vi "运维调试_CODCr.vi"() -> ()   [LabVIEW 2016, in "CodCr.lvlib"]
uses:
  CodCr.lvlib
  <vilib>/Utility/miscctls.llb/LVPointTypeDef.ctl
  <vilib>/Plasmionique/MB Master/MB_Master_Serial/MB_Master_Serial.lvclass
  C:/Program Files (x86)/National Instruments/LabVIEW 2016/vi.lib/Plasmionique/MB Master/MB_Master/MB_Master.lvclass
  <vilib>/Plasmionique/MB Master/MB Master.lvlib
  <vilib>/ptbypt/NI_PtbyPt.lvlib
panel:
  out "source":string
  in  "标样核查":bool
  out "启动时间":timestamp format="%<%Y/%m/%d %H:%M:%S>T"
  out "主循环次数":i32
  out "status":bool
  out "启动测量模式":T1(ring)
  out "曲线斜率B":sgl
  out "曲线斜率K":sgl
  out "量程上限":sgl
  out "量程下限":sgl
  out "消解时长":u16
  out "消解温度":u16
  out "测量精度":u16
  out "测量结果":sgl
  out "标样参考值":sgl
  out "量程":u16
  out "工作状态":T1(ring)
  out "仪器时间":timestamp format="%<%X\n%x>T"
  out "关键参数区":T2
  out "状态告警区":T3
  out "测量数据区":T4 {"单位" items=["ug/L", "mg/L", "ppm", "mg/m3", "cm", "ppb", "ug/m3", "%", "nmol/mol", "umol/mol", "MPN/L", "MPN/100ml", "ng/m3", "NTU", "无量纲", "ms/cm", "us/cm", "℃", "mV", "万个/L"]}
  out "系统时间":timestamp format="%<%Y/%m/%d %H:%M:%S>T"
  in  "VISA Resource":refnum<visa-resource-name>="COM9"
  out "Registers":u16[](array[numeric])
  in  "枚举":enum16{"读取", "写入", "读取参数"}(ring)
  in  "停止":bool
  in  "校时":bool
  in  "标样校准":bool
  in  "空白校准":bool
  in  "零点核查":bool
  in  "跨度核查":bool
  in  "水样测试":bool
  in  "返回":bool
  in  "设置":bool
  # "mg/L"
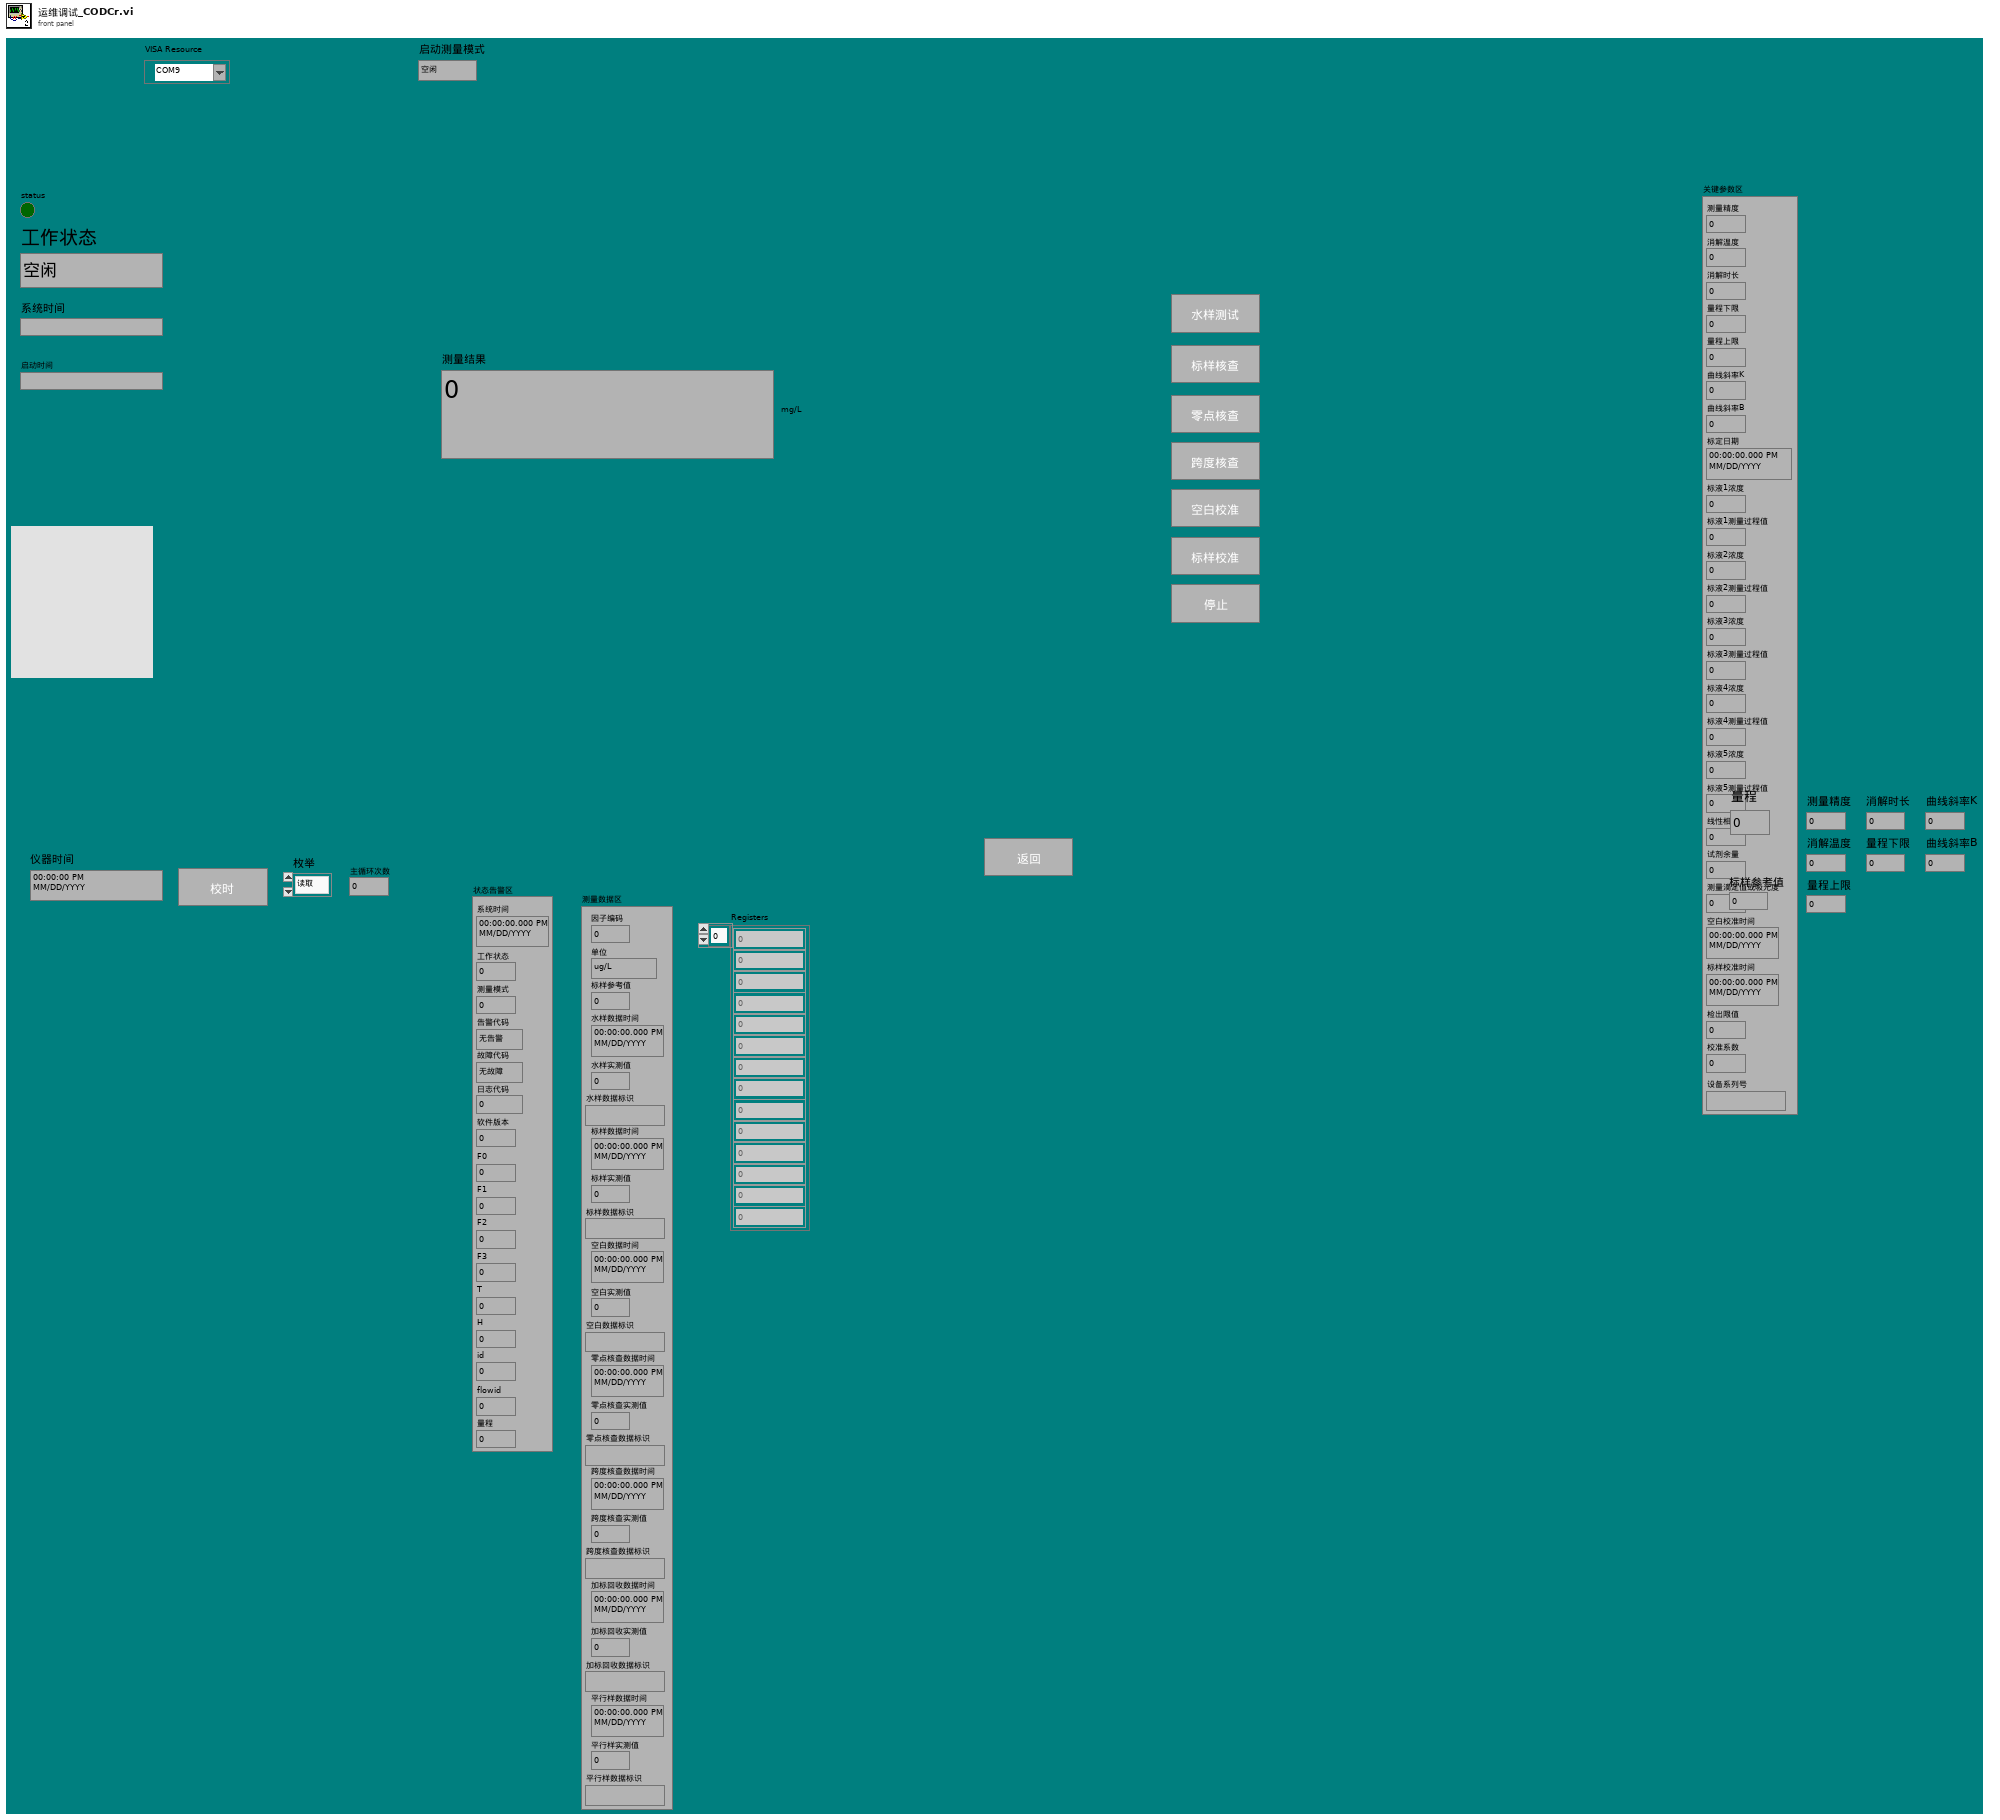
[diagram p1: front panel]
types:
  T1 = enum16{"空闲", "水样测试", "标样核查", "零点核查", "跨度核查", "空白测试", "平行样测试", "加标回收", "空白校准", "标样校准", "初始化（清洗）"}
  T2 = cluster{"测量精度":u16, "消解温度":u16, "消解时长":u16, "量程下限":sgl, "量程上限":sgl, "曲线斜率K":sgl, "曲线斜率B":sgl, "标定日期":timestamp, "标液1浓度":sgl, "标液1测量过程值":sgl, "标液2浓度":sgl, "标液2测量过程值":sgl, "标液3浓度":sgl, "标液3测量过程值":sgl, "标液4浓度":sgl, "标液4测量过程值":sgl, "标液5浓度":sgl, "标液5测量过程值":sgl, "线性相关系数":sgl, "试剂余量":u32, "测量滴定值或吸光度":sgl, "空白校准时间":timestamp, "标样校准时间":timestamp, "检出限值":sgl, "校准系数":sgl, "设备系列号":string}
  T3 = cluster{"系统时间":timestamp, "工作状态":u16, "测量模式":u16, "告警代码":enum16{"无告警", "缺试剂告警", "缺水样告警", "缺蒸馏水告警", "缺标液告警", "仪表漏液告警", "标定异常告警", "超量程告警", "加热异常", "低试剂预警", "超上限告警", "超下限告警", "仪表内部其他异常", "滴定异常告警", "电极异常告警", "量程切换告警", "参数设置告警", "PH电极电位异常", "电导率电极异常", "浊度光度异常", "溶解氧电极异常", "溶解氧光强异常", "温度异常告警", "PH异常告警", "溶解氧异常告警", "电导率异常告警", "浊度异常告警", "叶绿素异常告警", "藻密度异常告警", "蓝绿藻异常告警", "ORP异常告警", "氨氮异常告警", "清洁刷异常告警", "SD卡异常告警", "蓝牙异常告警", "Wifi异常告警", "流程异常告警"}, "故障代码":enum16{"无故障", "电机故障", "温度故障", "通讯故障", "滴定故障"}, "日志代码":u16, "软件版本":u16, "F0":sgl, "F1":sgl, "F2":sgl, "F3":sgl, "T":sgl, "H":sgl, "id":u16, "flowid":u16, "量程":u16}
  T4 = cluster{"因子编码":u32, "单位":u16, "标样参考值":sgl, "水样数据时间":timestamp, "水样实测值":sgl, "水样数据标识":string, "标样数据时间":timestamp, "标样实测值":sgl, "标样数据标识":string, "空白数据时间":timestamp, "空白实测值":sgl, "空白数据标识":string, "零点核查数据时间":timestamp, "零点核查实测值":sgl, "零点核查数据标识":string, "跨度核查数据时间":timestamp, "跨度核查实测值":sgl, "跨度核查数据标识":string, "加标回收数据时间":timestamp, "加标回收实测值":sgl, "加标回收数据标识":string, "平行样数据时间":timestamp, "平行样实测值":sgl, "平行样数据标识":string}
  T5 = cluster{"baud rate (bps)":u32, "stop bits":u16, "parity":u16, "flow control":u16, "timeout":u32, "retries":i32}
  T6 = cluster{"starting address":u16, "number of holding registers":u16}
  T7 = typedef "LVPointTypeDef.ctl" = cluster{"Horizontal":i16, "Vertical":i16}
  T8 = cluster{"时间标识":timestamp, "监测值":sgl, "单位":u16, "数据标识":string, "因子编码":u32, "标样参考值":sgl, "F0":sgl, "F1":sgl, "F2":sgl, "F3":sgl, "温度":sgl, "湿度":sgl, "量程标识":string}
  T9 = cluster{"系统时间":timestamp, "工作状态":enum16{"空闲", "水样测试", "标样核查", "零点核查", "跨度核查", "空白测试", "平行样测试", "加标回收", "空白校准", "标样校准", "初始化（清洗）"}, "测量模式":enum16{"待机", "连续模式", "周期模式", "定点模式", "受控模式", "手动模式"}, "告警代码":enum16{"无告警", "缺试剂告警", "缺水样告警", "缺蒸馏水告警", "缺标液告警", "仪表漏液告警", "标定异常告警", "超量程告警", "加热异常", "低试剂预警", "超上限告警", "超下限告警", "仪表内部其他异常", "滴定异常告警", "电极异常告警", "量程切换告警", "参数设置告警", "PH电极电位异常", "电导率电极异常", "浊度光度异常", "溶解氧电极异常", "溶解氧光强异常", "温度异常告警", "PH异常告警", "溶解氧异常告警", "电导率异常告警", "浊度异常告警", "叶绿素异常告警", "藻密度异常告警", "蓝绿藻异常告警", "ORP异常告警", "氨氮异常告警", "清洁刷异常告警", "SD卡异常告警", "蓝牙异常告警", "Wifi异常告警", "流程异常告警"}, "故障代码":enum16{"无故障", "电机故障", "温度故障", "通讯故障", "滴定故障"}, "日志代码":u16, "软件版本":u16, "F0":sgl, "F1":sgl, "F2":sgl, "F3":sgl, "T":sgl, "H":sgl, "id":u16, "flowid":u16, "量程":u16}
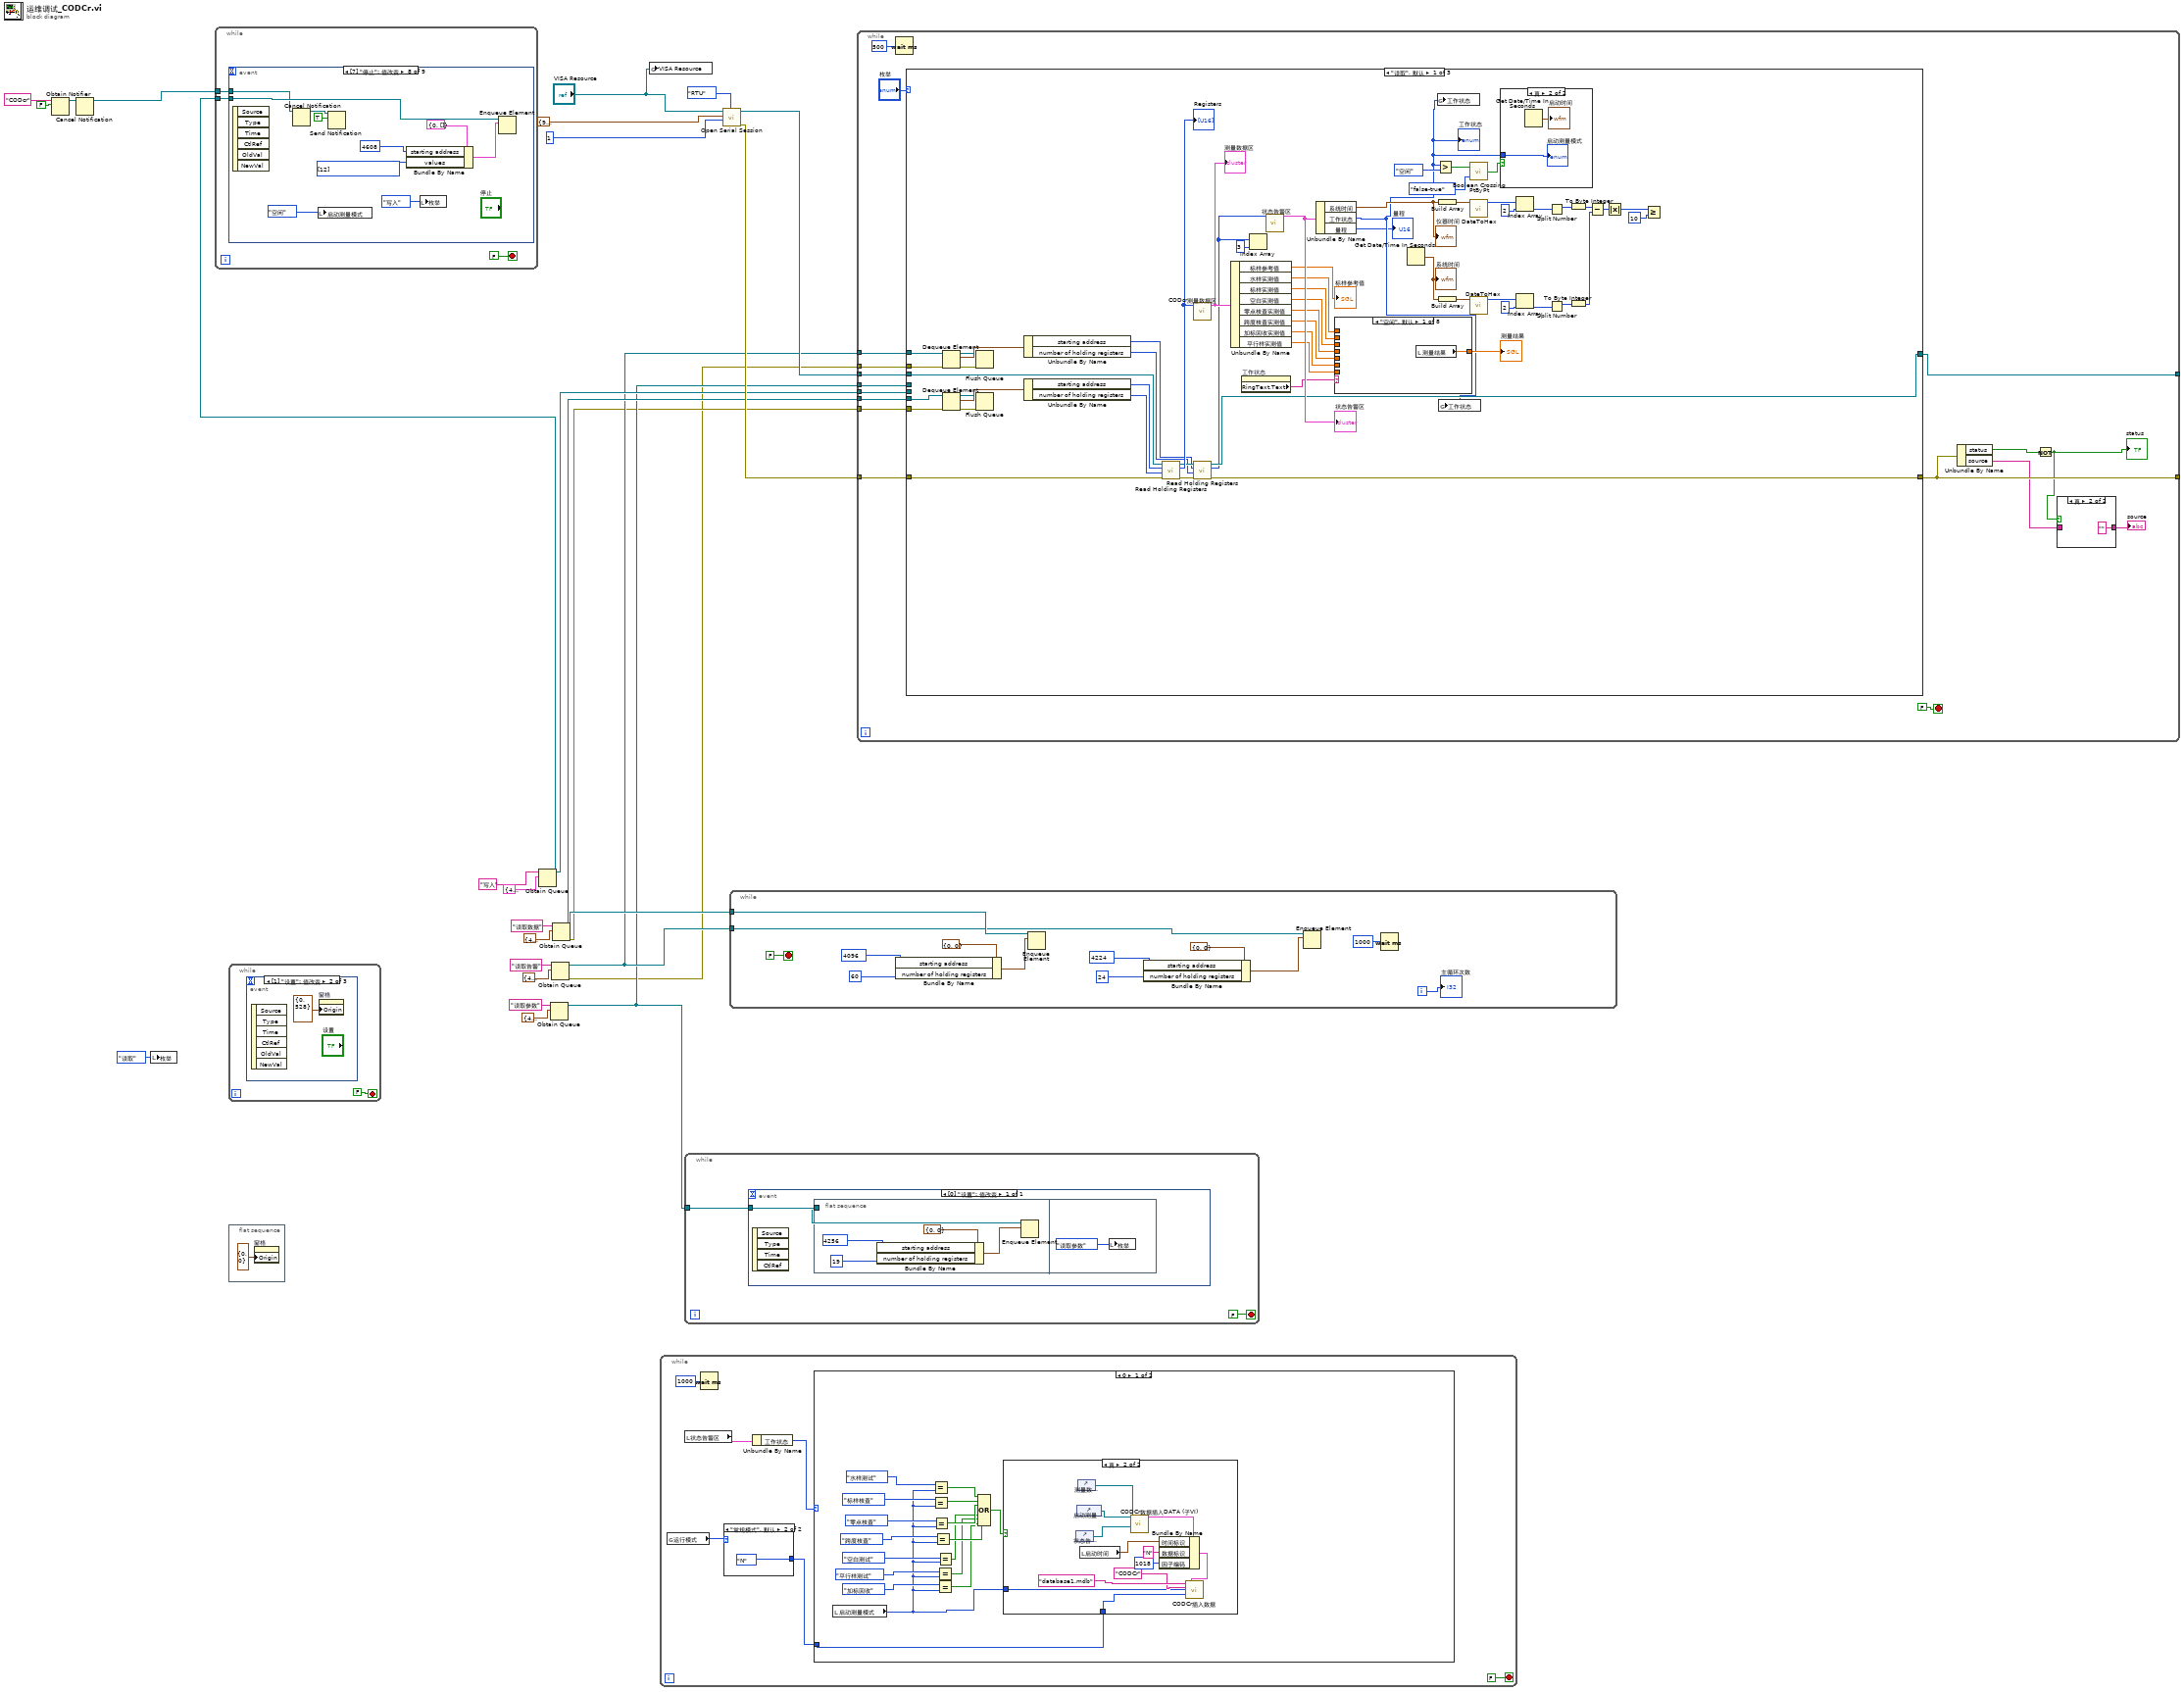
[diagram p0: block diagram]
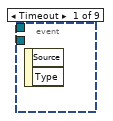
[diagram p2: hidden frame]
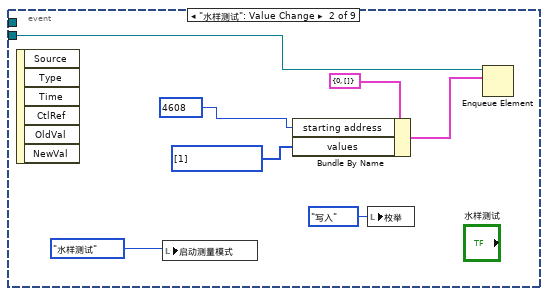
[diagram p3: hidden frame]
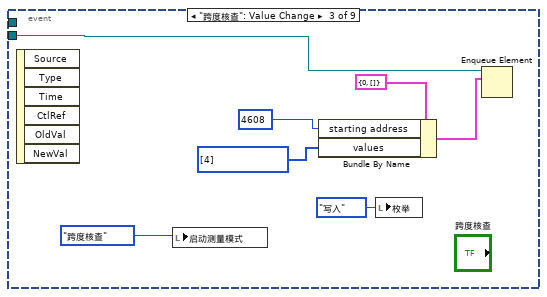
[diagram p4: hidden frame]
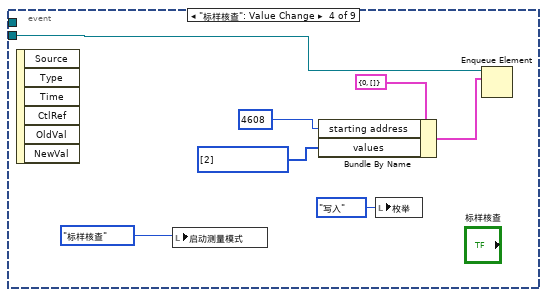
[diagram p5: hidden frame]
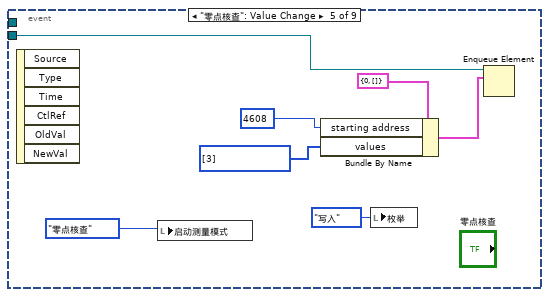
[diagram p6: hidden frame]
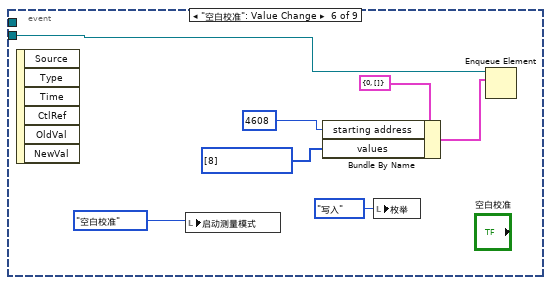
[diagram p7: hidden frame]
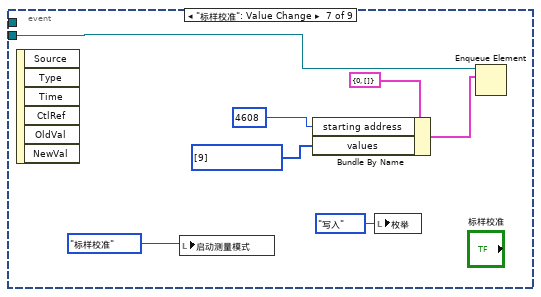
[diagram p8: hidden frame]
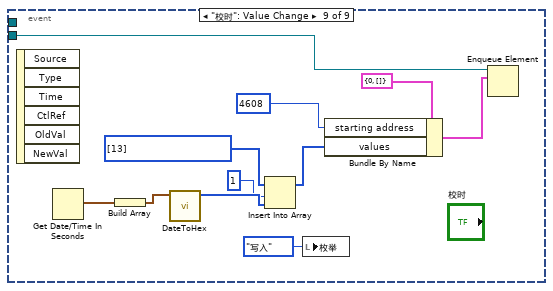
[diagram p9: hidden frame]
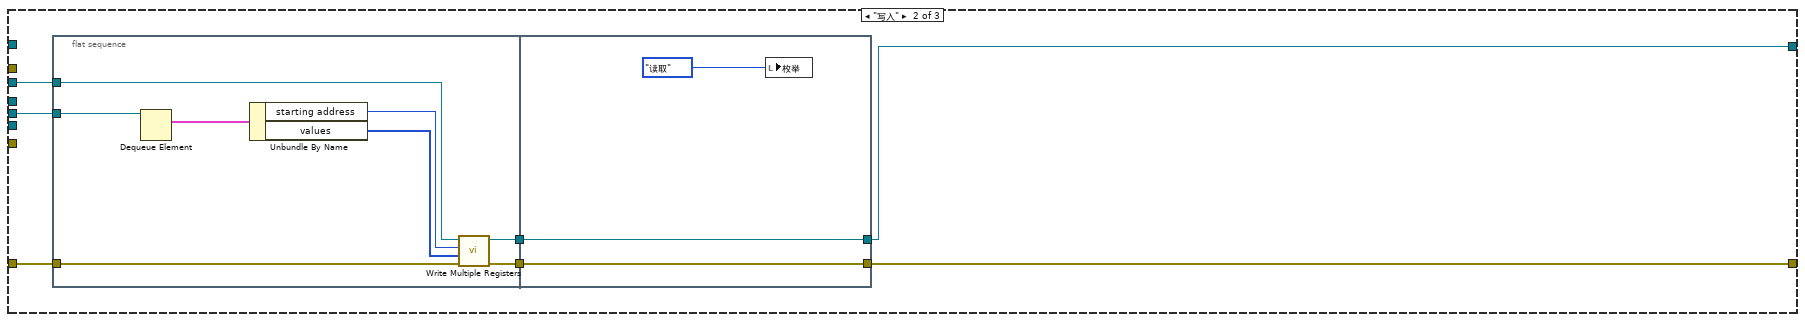
[diagram p19: hidden frame]
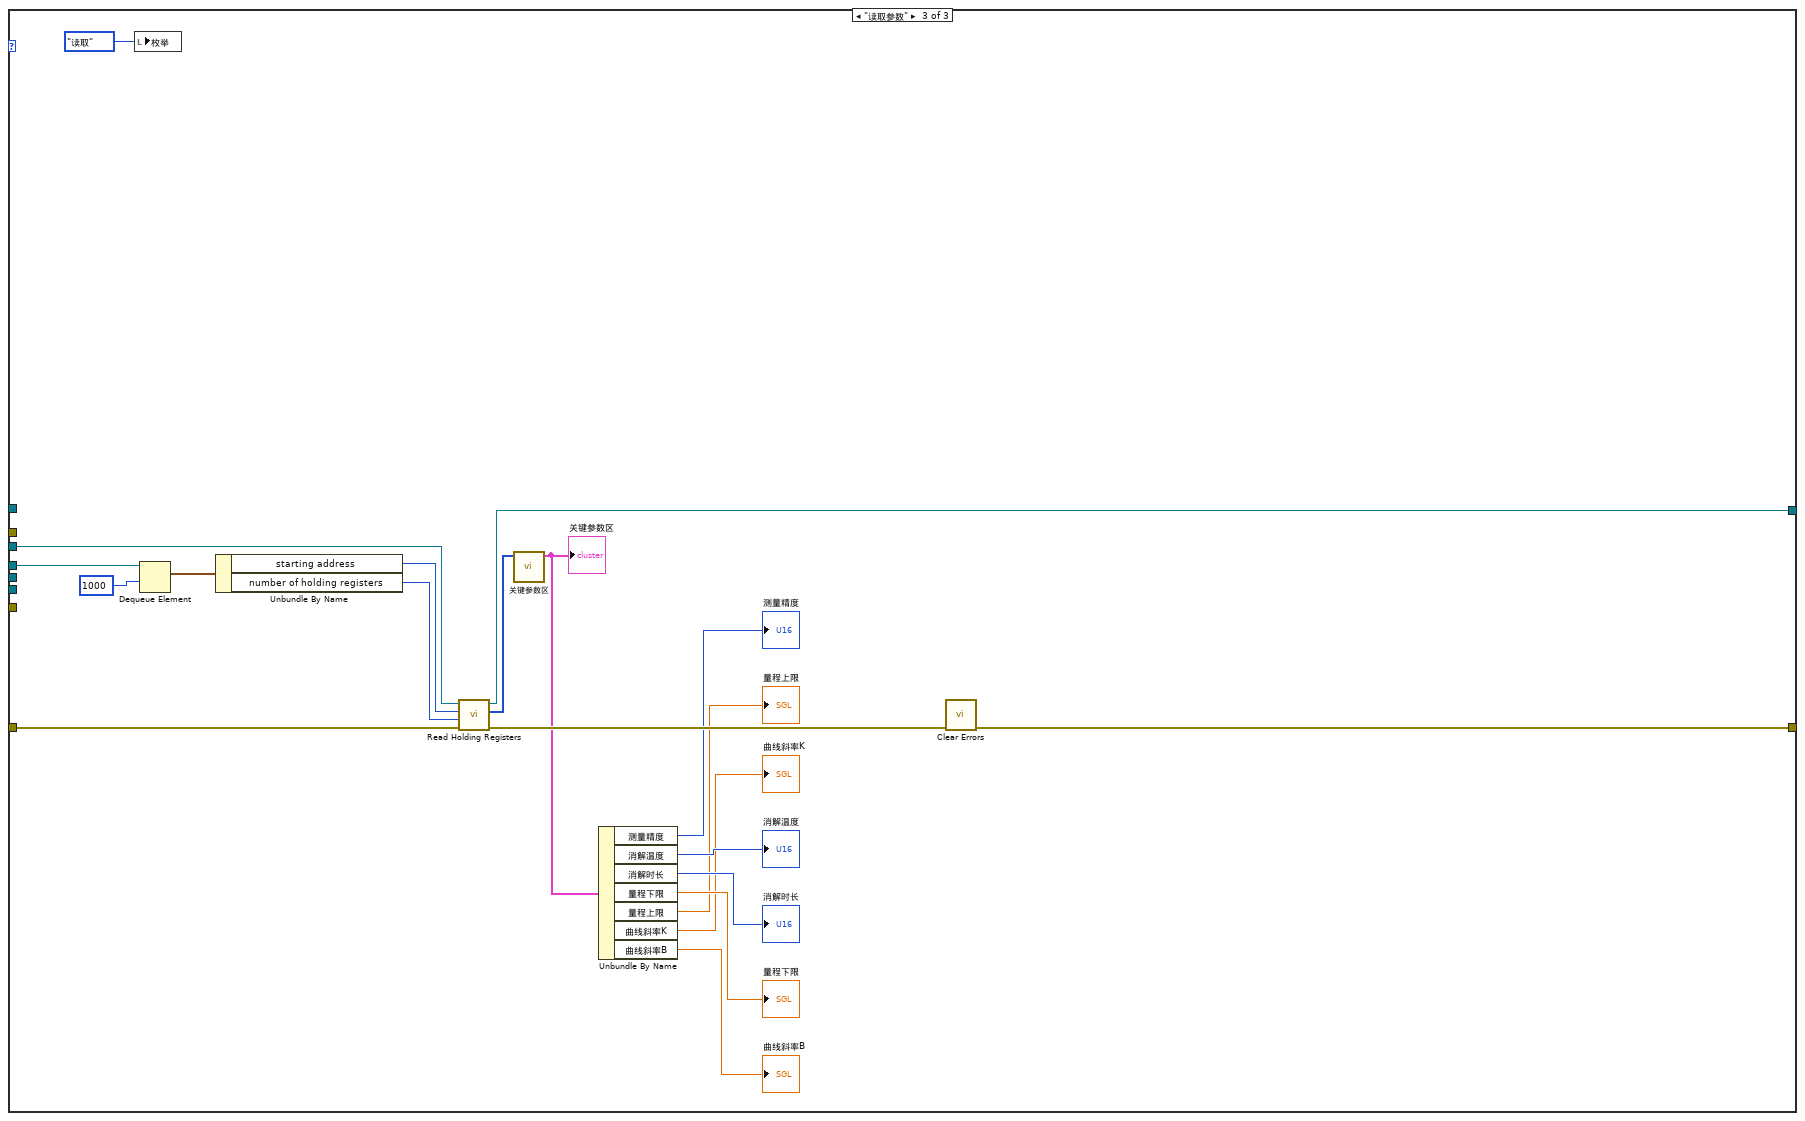
[diagram p20: hidden frame]
diagram:
  n1 = Obtain Notifier(name (unnamed)="CODcr" ("名称（未命名）"), notification data type=FALSE) -> (notifier out=w2:refnum<notifier>)  [unwired: 2 in, 2 out]
  n2 = Cancel Notification(0:w2) -> (8:w3:refnum<notifier>)  [unwired: 1 in, 2 out]
  n3 = local write "枚举"(enum16{"读取", "写入", "读取参数"}."读取" ("枚举")) -> ()
  n4 = while {
    stop <- FALSE stop-if-true
    n5 = event shown="[1] \"设置\": 值改变" {
      selector: _ -> [_ _ _]
      dyn-events: _ -> [_ _ _]
      timeout: _ -> [_ _ _]
      event Timeout {
        n6 = event-data() -> ()  [unwired: 1 in, 3 out]
      }
      event "设置": Value Change {
        n7 = event-data() -> ()  [unwired: 1 in, 6 out]
        n8 = property on="窗格" class="Pane"("Origin"=T7 {"Horizontal"=0, "Vertical"=528} ("原点")) -> ()  [unwired: 2 in, 2 out]
      }
      event "返回": Value Change {
        n9 = event-data() -> ()  [unwired: 1 in, 6 out]
        n10 = property on="窗格" class="Pane"("Origin"=T7 {"Horizontal"=0, "Vertical"=0} ("原点")) -> ()  [unwired: 2 in, 2 out]
      }
    }
  }
  n11 = flat-sequence {
    frame #0 {
      n12 = property on="窗格" class="Pane"("Origin"=T7 {"Horizontal"=0, "Vertical"=0} ("原点")) -> ()  [unwired: 2 in, 2 out]
    }
  }
  n13 = Obtain Queue(name (unnamed)="写入" ("名称（未命名）"), element data type=cluster{"starting address":u16, "values":u16[]} {"starting address"=4096, "values"=[]}) -> (queue out=w15:refnum<queue>)  [unwired: 3 in, 2 out]
  n14 = while {
    tunnel: w15 -> [w31]
    tunnel: w3 -> [w30]
    stop <- FALSE stop-if-true
    n15 = event shown="[7] \"停止\": 值改变" {
      selector: _ -> [_ _ _ _ _ _ _ _ _]
      dyn-events: _ -> [_ _ _ _ _ _ _ _ _]
      timeout: _ -> [_ _ _ _ _ _ _ _ _]
      tunnel: w31 -> [_ w39 w42 w49 w56 w63 w70 w80 w92]
      tunnel: w30 -> [_ _ _ _ _ _ _ w78 _]
      event Timeout {
        n16 = event-data() -> ()  [unwired: 1 in, 2 out]
      }
      event "水样测试": Value Change {
        n17 = event-data() -> ()  [unwired: 1 in, 6 out]
        n18 = local write "启动测量模式"(T1."水样测试" ("启动测量模式")) -> ()
        n19 = Bundle By Name(cluster=cluster{"starting address":u16, "values":u16[]} {"starting address"=0, "values"=[]} ("元素"), "starting address"=u16 4608, "values"=u16[] [1]) -> (w37:cluster{"starting address":u16, "values":u16[]})
        n20 = local write "枚举"(enum16{"读取", "写入", "读取参数"}."写入" ("枚举")) -> ()
        n21 = Enqueue Element(queue=w39, element=w37) -> ()  [unwired: 2 in, 3 out]
      }
      event "跨度核查": Value Change {
        n22 = event-data() -> ()  [unwired: 1 in, 6 out]
        n23 = local write "启动测量模式"(T1."跨度核查" ("启动测量模式")) -> ()
        n24 = Bundle By Name(cluster=cluster{"starting address":u16, "values":u16[]} {"starting address"=0, "values"=[]} ("元素"), "starting address"=u16 4608, "values"=u16[] [4]) -> (w45:cluster{"starting address":u16, "values":u16[]})
        n25 = local write "枚举"(enum16{"读取", "写入", "读取参数"}."写入" ("枚举")) -> ()
        n26 = Enqueue Element(queue=w42, element=w45) -> ()  [unwired: 2 in, 3 out]
      }
      event "标样核查": Value Change {
        n27 = event-data() -> ()  [unwired: 1 in, 6 out]
        n28 = local write "启动测量模式"(T1."标样核查" ("启动测量模式")) -> ()
        n29 = Bundle By Name(cluster=cluster{"starting address":u16, "values":u16[]} {"starting address"=0, "values"=[]} ("元素"), "starting address"=u16 4608, "values"=u16[] [2]) -> (w52:cluster{"starting address":u16, "values":u16[]})
        n30 = local write "枚举"(enum16{"读取", "写入", "读取参数"}."写入" ("枚举")) -> ()
        n31 = Enqueue Element(queue=w49, element=w52) -> ()  [unwired: 2 in, 3 out]
      }
      event "零点核查": Value Change {
        n32 = event-data() -> ()  [unwired: 1 in, 6 out]
        n33 = local write "启动测量模式"(T1."零点核查" ("启动测量模式")) -> ()
        n34 = Bundle By Name(cluster=cluster{"starting address":u16, "values":u16[]} {"starting address"=0, "values"=[]} ("元素"), "starting address"=u16 4608, "values"=u16[] [3]) -> (w59:cluster{"starting address":u16, "values":u16[]})
        n35 = local write "枚举"(enum16{"读取", "写入", "读取参数"}."写入" ("枚举")) -> ()
        n36 = Enqueue Element(queue=w56, element=w59) -> ()  [unwired: 2 in, 3 out]
      }
      event "空白校准": Value Change {
        n37 = event-data() -> ()  [unwired: 1 in, 6 out]
        n38 = local write "启动测量模式"(T1."空白校准" ("启动测量模式")) -> ()
        n39 = Bundle By Name(cluster=cluster{"starting address":u16, "values":u16[]} {"starting address"=0, "values"=[]} ("元素"), "starting address"=u16 4608, "values"=u16[] [8]) -> (w66:cluster{"starting address":u16, "values":u16[]})
        n40 = local write "枚举"(enum16{"读取", "写入", "读取参数"}."写入" ("枚举")) -> ()
        n41 = Enqueue Element(queue=w63, element=w66) -> ()  [unwired: 2 in, 3 out]
      }
      event "标样校准": Value Change {
        n42 = event-data() -> ()  [unwired: 1 in, 6 out]
        n43 = local write "启动测量模式"(T1."标样校准" ("启动测量模式")) -> ()
        n44 = Bundle By Name(cluster=cluster{"starting address":u16, "values":u16[]} {"starting address"=0, "values"=[]} ("元素"), "starting address"=u16 4608, "values"=u16[] [9]) -> (w73:cluster{"starting address":u16, "values":u16[]})
        n45 = local write "枚举"(enum16{"读取", "写入", "读取参数"}."写入" ("枚举")) -> ()
        n46 = Enqueue Element(queue=w70, element=w73) -> ()  [unwired: 2 in, 3 out]
      }
      event "停止": Value Change {
        n47 = event-data() -> ()  [unwired: 1 in, 6 out]
        n48 = Cancel Notification(0:w78) -> (8:w77:refnum<notifier>)  [unwired: 1 in, 2 out]
        n49 = local write "启动测量模式"(T1."空闲" ("启动测量模式")) -> ()
        n50 = Send Notification(notification=TRUE ("通知"), notifier=w77) -> ()  [unwired: 1 in, 2 out]
        n51 = Bundle By Name(cluster=cluster{"starting address":u16, "values":u16[]} {"starting address"=0, "values"=[]} ("元素"), "starting address"=u16 4608, "values"=u16[] [12]) -> (w83:cluster{"starting address":u16, "values":u16[]})
        n52 = local write "枚举"(enum16{"读取", "写入", "读取参数"}."写入" ("枚举")) -> ()
        n53 = Enqueue Element(queue=w80, element=w83) -> ()  [unwired: 2 in, 3 out]
      }
      event "校时": Value Change {
        n54 = event-data() -> ()  [unwired: 1 in, 6 out]
        n55 = Get Date/Time In Seconds() -> (seconds since 1Jan1904=w91:timestamp)
        n56 = Build Array(w91) -> (w90:timestamp[])
        n57 = call "DateToHex.vi"("DATE"=w90) -> ("数组"=w88:u16[])  [unwired: 10 in]
        n58 = Insert Into Array(array=u16[] [13] ("values"), index=1 ("索引"), new element=w88) -> (w86:u16[])
        n59 = local write "枚举"(enum16{"读取", "写入", "读取参数"}."写入" ("枚举")) -> ()
        n60 = Bundle By Name(cluster=cluster{"starting address":u16, "values":u16[]} {"starting address"=0, "values"=[]} ("元素"), "starting address"=u16 4608, "values"=w86) -> (w94:cluster{"starting address":u16, "values":u16[]})
        n61 = Enqueue Element(queue=w92, element=w94) -> ()  [unwired: 2 in, 3 out]
      }
    }
  }
  n62 = Obtain Queue(name (unnamed)="读取参数" ("名称（未命名）"), element data type=T6 {"starting address"=4096, "number of holding registers"=100}) -> (queue out=w9:refnum<queue>)  [unwired: 3 in, 2 out]
  n63 = Obtain Queue(name (unnamed)="读取告警" ("名称（未命名）"), element data type=T6 {"starting address"=4096, "number of holding registers"=100}) -> (queue out=w12:refnum<queue>, error out=w6:errorcluster)  [unwired: 3 in, 1 out]
  n64 = Obtain Queue(name (unnamed)="读取数据" ("名称（未命名）"), element data type=T6 {"starting address"=4096, "number of holding registers"=100}) -> (queue out=w16:refnum<queue>, error out=w7:errorcluster)  [unwired: 3 in, 1 out]
  n65 = global write "CODcr全局变量.vi" "VISA Resource"("VISA Resource") -> ()
  n66 = while {
    stop <- FALSE stop-if-true
    n67 = global read "系统变量.vi" "运行模式"() -> (w97:enum16{"维护模式", "常规模式", "应急模式", "质控模式"})
    n68 = local read "状态告警区"() -> (w99:T3)
    n69 = Wait (ms)(milliseconds to wait=u32 1000 ("等待时间（毫秒）")) -> ()  [unwired: 1 out]
    n70 = case shown="\"常规模式\", 默认" w97 {
      tunnel: [enum16{"N", "M"}."M" ("数据类型") enum16{"N", "M"}."N" ("数据类型")] -> w96
      frame "维护模式" {
      }
      frame "常规模式", Default {
      }
    }
    n71 = Unbundle By Name(w99) -> ("工作状态"=w98:u16)
    n72 = case shown="0" w98 {
      tunnel: w96 -> [w120 _]
      frame 0 {
        n73 = local read "启动测量模式"() -> (w112:T1)
        n74 = Equal?(x=T1."水样测试" ("启动测量模式"), y=w112) -> (x = y?=w111:bool)
        n75 = Equal?(x=T1."标样核查" ("启动测量模式"), y=w112) -> (x = y?=w110:bool)
        n76 = Equal?(x=T1."零点核查" ("启动测量模式"), y=w112) -> (x = y?=w109:bool)
        n77 = Equal?(x=T1."跨度核查" ("启动测量模式"), y=w112) -> (x = y?=w108:bool)
        n78 = Equal?(x=T1."平行样测试" ("启动测量模式"), y=w112) -> (x = y?=w106:bool)
        n79 = Equal?(x=T1."加标回收" ("启动测量模式"), y=w112) -> (x = y?=w105:bool)
        n80 = Equal?(x=T1."空白测试" ("启动测量模式"), y=w112) -> (x = y?=w107:bool)
        n81 = Compound Arithmetic op=OR(w111, w110, w109, w108, w107, w106, w105) -> (w104:bool)
        n82 = case shown="真" w104 {
          tunnel: w112 -> [_ w130]
          tunnel: w120 -> [_ w129]
          frame False {
          }
          frame True {
            n83 = control-ref of="状态告警区"() -> (w126:refnum<vi>)
            n84 = control-ref of="启动测量模式"() -> (w128:refnum<vi>)
            n85 = control-ref of="测量数据区"() -> (w127:refnum<vi>)
            n86 = local read "启动时间"() -> (w124:timestamp)
            n87 = call "CODCr数据插入DATA (子VI).vi"("reference 2"=w126, "reference"=w127, "Enum输入"=w128) -> ("data"=w125:T8)  [unwired: 8 in]
            n88 = Bundle By Name(cluster=w125, "时间标识"=w124, "数据标识"="N", "因子编码"=u32 1018) -> (w123:T8)
            n89 = call "CODCr插入数据.vi"("database"="database1.mdb", "data"=w123, "table"="CODCr", "测量模式"=w130, "数据类型"=w129) -> ()  [unwired: 10 in, 1 out]
          }
        }
      }
      frame 1, Default {
      }
    }
  }
  n90 = while {
    tunnel: w9 -> [w133]
    stop <- FALSE stop-if-true
    n91 = event shown="[0] \"设置\": 值改变" {
      selector: _ -> [_]
      dyn-events: _ -> [_]
      timeout: _ -> [_]
      tunnel: w133 -> [w135]
      event "设置": Value Change {
        n92 = event-data() -> ()  [unwired: 1 in, 4 out]
        n93 = flat-sequence {
          tunnel: w135 -> [w136]
          frame #0 {
            n94 = Bundle By Name(cluster=T6 {"starting address"=0, "number of holding registers"=0} ("元素"), "starting address"=u16 4256, "number of holding registers"=u16 19) -> (w140:T6)
            n95 = Enqueue Element(queue=w136, element=w140) -> ()  [unwired: 2 in, 3 out]
          }
          frame #1 {
            n96 = local write "枚举"(enum16{"读取", "写入", "读取参数"}."读取参数" ("枚举")) -> ()
          }
        }
      }
    }
  }
  n97 = call <vilib>:"Open Serial Session.vi"("Mode (RTU)"=enum16{"RTU", "ASCII"}."RTU", "Slave ID"=u8 1, "Serial Config"=T5 {"baud rate (bps)"=9600, "stop bits"=10, "parity"=0, "flow control"=0, "timeout"=1000, "retries"=1}, "VISA Resource"="VISA Resource") -> ("Error out"=w24:errorcluster, "MB_Serial session"=w25:refnum<class "MB_Master_Serial.lvclass">)  [unwired: 6 in]
  n98 = while {
    tunnel: w16 -> [w152]
    tunnel: w12 -> [w143]
    i -> [w142]
    stop <- FALSE stop-if-true
    n99 = Bundle By Name(cluster=T6 {"starting address"=0, "number of holding registers"=0} ("元素"), "starting address"=u16 4096, "number of holding registers"=u16 60) -> (w150:T6)
    n100 = Enqueue Element(queue=w152, element=w150) -> ()  [unwired: 2 in, 3 out]
    n101 = Bundle By Name(cluster=T6 {"starting address"=0, "number of holding registers"=0} ("元素"), "starting address"=u16 4224, "number of holding registers"=u16 24) -> (w144:T6)
    n102 = Enqueue Element(queue=w143, element=w144) -> ()  [unwired: 2 in, 3 out]
    n103 = Wait (ms)(milliseconds to wait=u32 1000 ("等待时间（毫秒）")) -> ()  [unwired: 1 out]
    "主循环次数" <- w142
  }
  n104 = while {
    tunnel: w15 -> [w168]
    tunnel: w16 -> [w167]
    tunnel: w12 -> [w166]
    tunnel: w9 -> [w165]
    tunnel: w7 -> [w163]
    tunnel: w6 -> [w162]
    tunnel: w24 -> [w161]
    tunnel: [w159] -> _
    tunnel: w25 -> [w169]
    tunnel: [w164] -> _
    stop <- FALSE stop-if-true
    n105 = Wait (ms)(milliseconds to wait=u32 500 ("等待时间（毫秒）")) -> ()  [unwired: 1 out]
    n106 = case shown="\"读取\", 默认" "枚举" {
      tunnel: w169 -> [w231 w248 w271]
      tunnel: w161 -> [w206 w247 w270]
      tunnel: w168 -> [_ w246 _]
      tunnel: w167 -> [w230 _ _]
      tunnel: w166 -> [w225 _ _]
      tunnel: w165 -> [_ _ w272]
      tunnel: [w205 w242 w260] -> w159
      tunnel: [w187 w243 w261] -> w164
      tunnel: w163 -> [w181 _ _]
      tunnel: w162 -> [w178 _ _]
      frame "读取", Default {
        n107 = Dequeue Element(queue=w225, error in (no error)=w178) -> (queue out=w180:refnum<queue>, element=w224:T6, error out=w179:errorcluster)  [unwired: 1 in, 1 out]
        n108 = Dequeue Element(queue=w230, error in (no error)=w181) -> (queue out=w183:refnum<queue>, element=w229:T6, error out=w182:errorcluster)  [unwired: 1 in, 1 out]
        n109 = Flush Queue(queue=w180, error in (no error)=w179) -> ()  [unwired: 3 out]
        n110 = Flush Queue(queue=w183, error in (no error)=w182) -> ()  [unwired: 3 out]
        n111 = Unbundle By Name(w224) -> ("starting address"=w221:u16, "number of holding registers"=w220:u16)
        n112 = Unbundle By Name(w229) -> ("starting address"=w228:u16, "number of holding registers"=w227:u16)
        n113 = call <vilib>:"Read Holding Registers.vi"("error in (no error)"=w206, "quantity"=w227, "starting address"=w228, "MB session in"=w231) -> ("error out"=w222:errorcluster, "Registers"=w226:u16[], "MB session out"=w223:refnum<class "MB_Master_Serial.lvclass">)  [unwired: 5 in]
        "Registers" <- w226
        n114 = call "CODcr测量数据区.vi"("数组"=w226) -> ("测量数据区"=w218:T4)  [unwired: 10 in]
        "测量数据区" <- w218
        n115 = call <vilib>:"Read Holding Registers.vi"("error in (no error)"=w222, "quantity"=w220, "starting address"=w221, "MB session in"=w223) -> ("error out"=w205:errorcluster, "Registers"=w177:u16[], "MB session out"=w187:refnum<class "MB_Master_Serial.lvclass">)  [unwired: 5 in]
        n116 = Unbundle By Name(w218) -> ("标样参考值"=→"标样参考值":sgl, "水样实测值"=w214:sgl, "标样实测值"=w212:sgl, "空白实测值"=w209:sgl, "零点核查实测值"=w211:sgl, "跨度核查实测值"=w210:sgl, "加标回收实测值"=w207:sgl, "平行样实测值"=w208:sgl)
        n117 = property on="工作状态" class="Enum (严格)"() -> ("RingText.Text"=w215:string)  [unwired: 2 in, 2 out]
        n118 = Index Array(array=w177, index=3 ("索引")) -> ()  [unwired: 1 out]
        n119 = call "状态告警区.vi"("数组"=w177) -> ("状态告警区"=w219:T9)  [unwired: 10 in]
        "状态告警区" <- w219
        n120 = Unbundle By Name(w219) -> ("系统时间"=w188:timestamp, "工作状态"=w175:T1, "量程"=→"量程":u16)
        "仪器时间" <- w188
        "工作状态" <- w175
        n121 = case shown="\"空闲\", 默认" w215 {
          tunnel: w214 -> [_ w233 _ _ _ _ _ _]
          tunnel: [w232 w233 w234 w235 w236 w237 w238 w239] -> w213
          tunnel: w212 -> [_ _ w234 _ _ _ _ _]
          tunnel: w211 -> [_ _ _ w235 _ _ _ _]
          tunnel: w210 -> [_ _ _ _ w236 _ _ _]
          tunnel: w209 -> [_ _ _ _ _ w237 _ _]
          tunnel: w208 -> [_ _ _ _ _ _ w238 _]
          tunnel: w207 -> [_ _ _ _ _ _ _ w239]
          frame "空闲", Default {
            n122 = local read "测量结果"() -> (w232:sgl)
          }
          frame "水样测试" {
          }
          frame "标样核查" {
          }
          frame "零点核查" {
          }
          frame "跨度核查" {
          }
          frame "空白测试" {
          }
          frame "平行样测试" {
          }
          frame "加标回收" {
          }
        }
        "测量结果" <- w213
        n123 = Get Date/Time In Seconds() -> (seconds since 1Jan1904=w190:timestamp)
        "系统时间" <- w190
        n124 = Greater?(x=w175, y=T1."空闲") -> (0:w186:bool)
        n125 = global write "CODcr全局变量.vi" "工作状态"(w175) -> ()
        n126 = Build Array(w188) -> (w204:timestamp[])
        n127 = Build Array(w190) -> (w189:timestamp[])
        n128 = global write "CODCr工作状态.vi" "工作状态"(w175) -> ()
        n129 = call <vilib>:"Boolean Crossing PtByPt.vi"("direction"=enum16{"either", "false-true", "true-false"}."false-true", "input"=w186) -> ("crossing"=w185:bool)  [unwired: 1 in]
        n130 = call "DateToHex.vi"("DATE"=w204) -> ("数组"=w196:u16[])  [unwired: 10 in]
        n131 = call "DateToHex.vi"("DATE"=w189) -> ("数组"=w191:u16[])  [unwired: 10 in]
        n132 = case shown="真" w185 {
          tunnel: w175 -> [_ w240]
          frame False {
          }
          frame True {
            n133 = Get Date/Time In Seconds() -> (seconds since 1Jan1904=→"启动时间":timestamp)
            "启动测量模式" <- w240
          }
        }
        n134 = Index Array(array=w196, index=2 ("索引")) -> (element=w194:u16)
        n135 = Index Array(array=w191, index=2 ("索引")) -> (element=w193:u16)
        n136 = Split Number(x=w194) -> (hi(x)=w200:u8)  [unwired: 1 out]
        n137 = Split Number(x=w193) -> (hi(x)=w197:u8)  [unwired: 1 out]
        n138 = To Byte Integer(number=w200) -> (8bit integer=w201:i8)
        n139 = To Byte Integer(number=w197) -> (8bit integer=w198:i8)
        n140 = Subtract(x=w201, y=w198) -> (x-y=w199:i8)
        n141 = Absolute Value(x=w199) -> (abs(x)=w202:i8)
        n142 = Greater Or Equal?(x=w202, y=i8 10) -> ()  [unwired: 1 out]
      }
      frame "写入" {
        n143 = flat-sequence {
          tunnel: w248 -> [w256]
          tunnel: w247 -> [w255]
          tunnel: w246 -> [w252]
          tunnel: [w254] -> w245
          tunnel: [w253] -> w244
          tunnel: w245 -> [w258]
          tunnel: w244 -> [w257]
          tunnel: [w258] -> w243
          tunnel: [w257] -> w242
          frame #0 {
            n144 = Dequeue Element(queue=w252) -> (element=w251:cluster{"starting address":u16, "values":u16[]})  [unwired: 2 in, 3 out]
            n145 = Unbundle By Name(w251) -> ("starting address"=w250:u16, "values"=w249:u16[])
            n146 = call <vilib>:"Write Multiple Registers.vi"("error in (no error)"=w255, "values"=w249, "starting address"=w250, "MB session in"=w256) -> ("error out"=w253:errorcluster, "MB session out"=w254:refnum<class "MB_Master_Serial.lvclass">)  [unwired: 6 in]
          }
          frame #1 {
            n147 = local write "枚举"(enum16{"读取", "写入", "读取参数"}."读取" ("枚举")) -> ()
          }
        }
      }
      frame "读取参数" {
        n148 = local write "枚举"(enum16{"读取", "写入", "读取参数"}."读取" ("枚举")) -> ()
        n149 = Dequeue Element(queue=w272, timeout in ms (-1)=1000 ("超时毫秒(-1)")) -> (element=w279:T6)  [unwired: 1 in, 3 out]
        n150 = Unbundle By Name(w279) -> ("starting address"=w278:u16, "number of holding registers"=w277:u16)
        n151 = call <vilib>:"Read Holding Registers.vi"("error in (no error)"=w270, "quantity"=w277, "starting address"=w278, "MB session in"=w271) -> ("error out"=w274:errorcluster, "Registers"=w276:u16[], "MB session out"=w261:refnum<class "MB_Master_Serial.lvclass">)  [unwired: 5 in]
        n152 = call "关键参数区.vi"("数组"=w276) -> ("关键参数区"=w273:T2)  [unwired: 10 in]
        "关键参数区" <- w273
        n153 = Unbundle By Name(w273) -> ("测量精度"=→"测量精度":u16, "消解温度"=→"消解温度":u16, "消解时长"=→"消解时长":u16, "量程下限"=→"量程下限":sgl, "量程上限"=→"量程上限":sgl, "曲线斜率K"=→"曲线斜率K":sgl, "曲线斜率B"=→"曲线斜率B":sgl)
        n154 = call <vilib>:"Clear Errors.vi"("error in (no error)"=w274) -> ("error out"=w260:errorcluster)  [unwired: 5 in, 1 out]
      }
    }
    n155 = Unbundle By Name(w159) -> ("status"=w160:bool, "source"=w157:string)
    n156 = Not(x=w160) -> (.not. x?=w156:bool)
    "status" <- w156
    n157 = case shown="真" w156 {
      tunnel: w157 -> [w172 _]
      tunnel: [w172 "" ("source")] -> w155
      frame False {
      }
      frame True {
      }
    }
    "source" <- w155
  }
